vi "MKS_PDR2000_read_set_points.vi"(8 "error in (no error)":errorcluster, 11 "PDR2000 COM port":refnum<visa-resource-name>) -> (0 "error out":errorcluster, 3 "PDR2000 COM port out":refnum<visa-resource-name>)   [LabVIEW 2019]
panel:
  out "Set point 2":dbl
  out "Set point 1":dbl
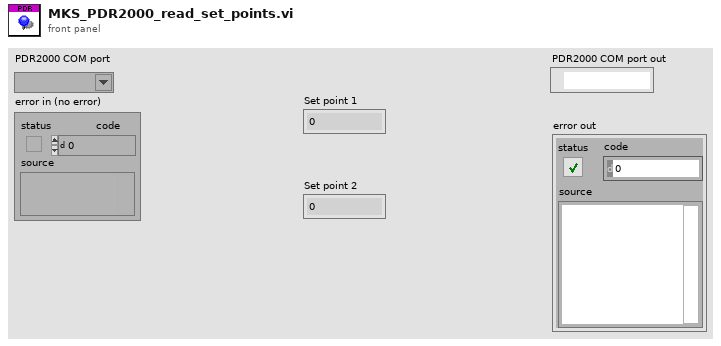
[diagram p1: front panel]
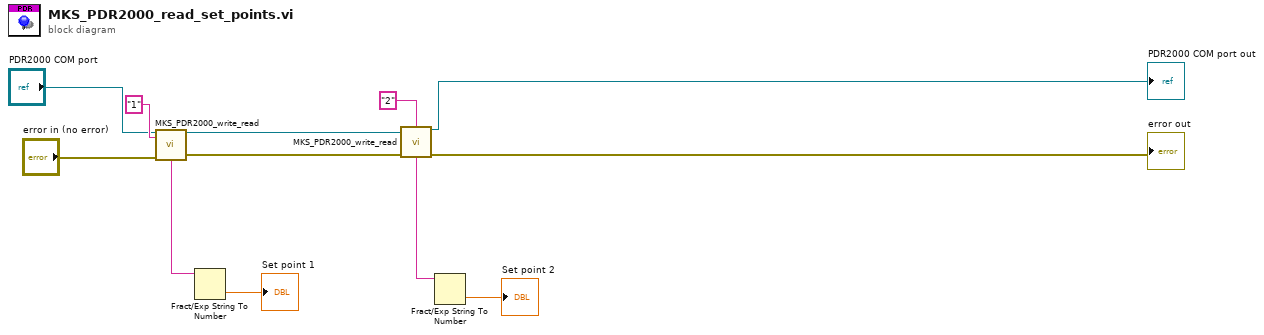
[diagram p0: block diagram]
diagram:
  n1 = call "MKS_PDR2000_write_read.vi"("PDR2000 COM port"="PDR2000 COM port", "Write string"="1", "error in (no error)"="error in (no error)") -> ("PDR2000 COM port out"=w9:refnum<visa-resource-name>, "Read String"=w5:string, "error out"=w8:errorcluster)  [unwired: 10 in]
  n2 = Fract/Exp String To Number(string=w5) -> (number=→"Set point 1":dbl)  [unwired: 3 in, 1 out]
  n3 = call "MKS_PDR2000_write_read.vi"("PDR2000 COM port"=w9, "Write string"="2", "error in (no error)"=w8) -> ("PDR2000 COM port out"=→"PDR2000 COM port out":refnum<visa-resource-name>, "Read String"=w3:string, "error out"=→"error out":errorcluster)  [unwired: 10 in]
  n4 = Fract/Exp String To Number(string=w3) -> (number=→"Set point 2":dbl)  [unwired: 3 in, 1 out]
